vi "Rotate Lockin Phase.vi"(9 "Phase":dbl(slide)=67.07142639160156 step=0.5 scale=-180.0..180.0, 10 "Array Y in":dbl[](array[numeric]) format="%.2f", 11 "Array X in":dbl[](array[numeric]) format="%.2f") -> (2 "Array Y out":dbl[](array[numeric]) format="%.2f", 3 "Array X out":dbl[](array[numeric]) format="%.2f")   [LabVIEW 2016]
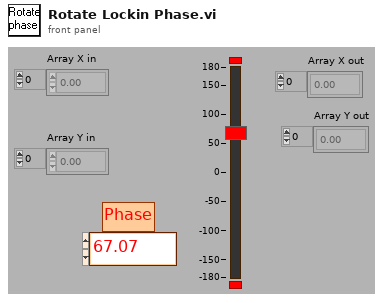
[diagram p1: front panel]
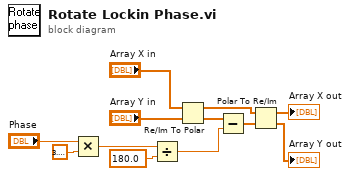
[diagram p0: block diagram]
diagram:
  n1 = Multiply(x="Phase", y=3.141592653589793) -> (x*y=w10:dbl)
  n2 = Divide(x=w10, y=180.0) -> (x/y=w12:dbl)
  n3 = Re/Im To Polar(2:"Array Y in", 3:"Array X in") -> (0:w6:dbl[], 1:w4:dbl[])
  n4 = Subtract(x=w6, y=w12) -> (x-y=w1:dbl[])
  n5 = Polar To Re/Im(2:w1, 3:w4) -> (0:→"Array Y out":dbl[], 1:→"Array X out":dbl[])
